vi "mod_IQ Impairments Frequency Offset.vi"(0 "Input Complex Waveform":T1 {"Y" format="%.3f"; "dt" format="%^.2e"; "t0" format="%.4f"}, 2 "Frequency Offset, Hz":dbl format="%.2f", 11 "error in (no error)":errorcluster, 13 "Reset? (T)":bool=TRUE) -> (4 "Output Complex Waveform":T1 {"Y" format="%.3f"; "dt" format="%^.2e"; "t0" format="%.4f"}, 15 "error out":errorcluster)   [LabVIEW 2020, in "niDMT.lvlib"]
doc: "Performs the Frequency Offset operation for IQ Impairment of an Input Data Waveform."
uses:
  <vilib>/addons/Modulation/niDMT.lvlib
  <vilib>/addons/Modulation/Analog/controls/Complex Data Waveform.ctl
  <vilib>/addons/Modulation/Digital/Support/Common/mod_Apply Frequency Offset (Internal).vi
  <vilib>/addons/Modulation/niAMT.lvlib
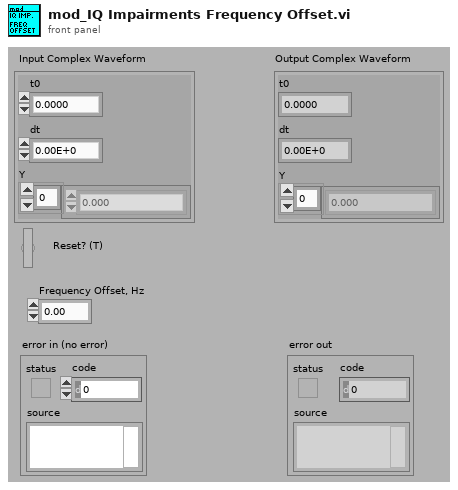
[diagram p1: front panel]
types:
  T1 = typedef "niAMT.lvlib/Complex Data Waveform.ctl" = cluster{"t0":dbl, "dt":dbl, "Y":cdb[]}
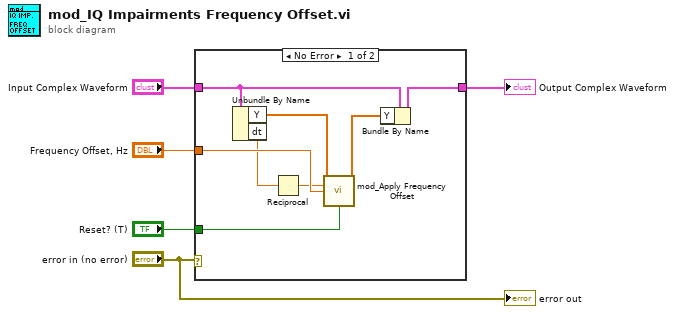
[diagram p0: block diagram]
diagram:
  n1 = case shown="No Error" "error in (no error)" {
    tunnel: "Reset? (T)" -> [w9 _]
    tunnel: "Input Complex Waveform" -> [w13 w14]
    tunnel: [w12 w14] -> w2
    tunnel: "Frequency Offset, Hz" -> [w8 _]
    frame No Error {
      n2 = Unbundle By Name(w13) -> ("Y"=w10:cdb[], "dt"=w6:dbl)
      n3 = Reciprocal(x=w6) -> (1/x=w7:dbl)
      n4 = call <vilib>:"mod_Apply Frequency Offset.vi"("Signal In"=w10, "Rate, pts/sec"=w7, "Freq Offset, Hz"=w8, "Reset? (T)"=w9) -> ("Signal Out"=w11:cdb[])  [unwired: 1 in, 10 out]
      n5 = Bundle By Name(cluster=w13, "Y"=w11) -> (w12:T1)
    }
    frame Error {
    }
  }
  "Output Complex Waveform" <- w2
  "error out" <- "error in (no error)"
